vi "detector-exposuretime-set.vi"(3 "Input Exposure Time":sgl format="%.2f") -> (0 "exp time ok":bool, 1 "Output Expsure Time":sgl format="%.2f")   [LabVIEW 2015]
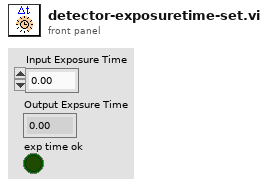
[diagram p1: front panel]
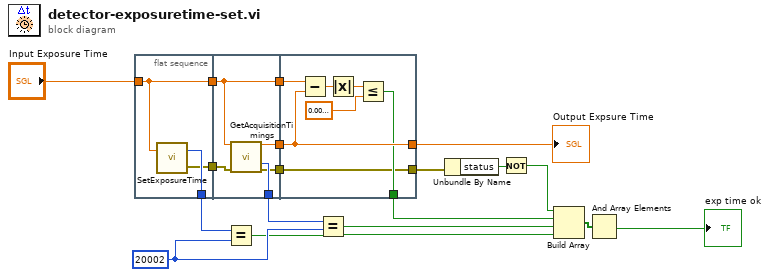
[diagram p0: block diagram]
diagram:
  w11 = u32 20002 ("= temperature\naccepted")
  n1 = flat-sequence {
    tunnel: "Input Exposure Time" -> [w21]
    tunnel: [w21] -> w17
    tunnel: [w20] -> w13
    tunnel: [w19] -> w5
    tunnel: w17 -> [w25]
    tunnel: [w25] -> w16
    tunnel: [w26] -> w15
    tunnel: [w24] -> w12
    tunnel: w5 -> [w23]
    tunnel: [w22] -> w4
    tunnel: w16 -> [w32]
    tunnel: w15 -> [w31]
    tunnel: [w28] -> w10
    tunnel: [w31] -> w14
    tunnel: [w27] -> w3
    tunnel: w4 -> [w27]
    frame #0 {
      n2 = call <userlib>:"SetExposureTime.vi"("time"=w21) -> ("error out"=w19:errorcluster, "DLL error code"=w20:u32)  [unwired: 1 in]
    }
    frame #1 {
      n3 = call <userlib>:"GetAcquisitionTimings.vi"("exposure input"=w25, "error in (no error)"=w23) -> ("exposure"=w26:sgl, "DLL error code"=w24:u32, "error out"=w22:errorcluster)  [unwired: 9 in, 2 out]
    }
    frame #2 {
      n4 = Subtract(x=w32, y=w31) -> (x-y=w33:sgl)
      n5 = Absolute Value(x=w33) -> (abs(x)=w30:sgl)
      n6 = Less Or Equal?(x=w30, y=sgl 0.01) -> (x <= y?=w28:bool)
    }
  }
  n7 = Equal?(x=w13, y=w11) -> (x = y?=w8:bool)
  n8 = Equal?(x=w12, y=w11) -> (x = y?=w9:bool)
  n9 = Unbundle By Name(w3) -> ("status"=w2:bool)
  n10 = Not(x=w2) -> (.not. x?=w1:bool)
  n11 = Build Array(w1, w10, w9, w8) -> (w7:bool[])
  n12 = And Array Elements(Boolean array=w7) -> (logical AND=→"exp time ok":bool)
  "Output Expsure Time" <- w14
